vi "Init_Calculation.vi"(8 "Tester Parameter":dbl[](array[numeric]), 9 "DDM Parameter":dbl[](array[numeric])) -> (2 "Data":dbl[](array[numeric]))   [LabVIEW 2017]
panel:
  out "voltage":dbl
  out "current":dbl
  out "power":dbl
  out "Ambient pressure":dbl
  out "Ambient temperature":dbl
  out "Ambient humidity":dbl
  out "pressure":dbl
  out "power":dbl
  out "speed":dbl
  out "power":dbl
  out "current":dbl
  out "voltage":dbl
  out "delta_v":dbl
  out "ddm real power":dbl
  out "DDM_Pressure corrected":dbl
  # "Suction Power at Rated Power [AW]"
  # "Measured Volumetric Flow Rate (Q)"
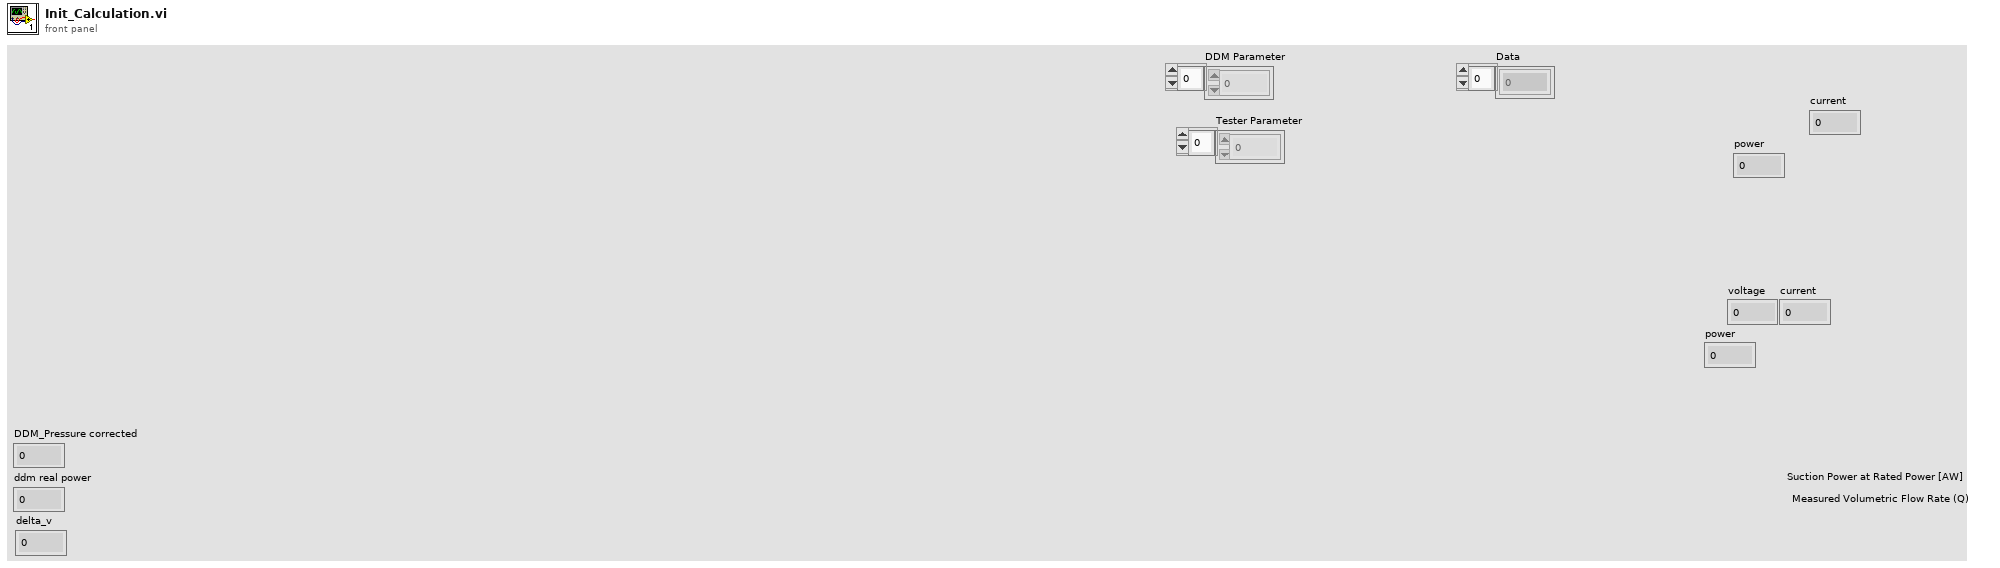
[diagram p1: front panel]
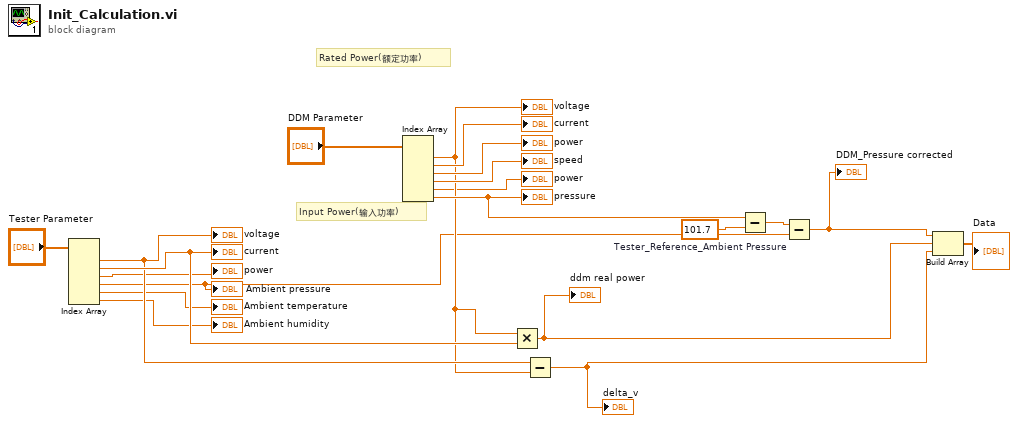
[diagram p0: block diagram]
diagram:
  w20 = 101.7  # Tester_Reference_Ambient Pressure
  # "Input Power(输入功率)"
  # "Rated Power(额定功率)"
  n1 = Index Array(array="Tester Parameter") -> (element #1=w11:dbl, element #2=w12:dbl, element #3=→"power":dbl, element #4=w9:dbl, element #5=→"Ambient temperature":dbl, element #6=→"Ambient humidity":dbl)  [unwired: 6 in]
  "voltage" <- w11
  "current" <- w12
  "Ambient pressure" <- w9
  n2 = Index Array(array="DDM Parameter") -> (element #1=w10:dbl, element #2=→"current":dbl, element #3=→"power":dbl, element #4=→"speed":dbl, element #5=→"power":dbl, element #6=w13:dbl)  [unwired: 6 in]
  "voltage" <- w10
  "pressure" <- w13
  n3 = Multiply(x=w10, y=w12) -> (x*y=w3:dbl)
  "ddm real power" <- w3
  n4 = Subtract(x=w11, y=w10) -> (x-y=w2:dbl)
  "delta_v" <- w2
  n5 = Subtract(x=w13, y=w20) -> (x-y=w19:dbl)
  n6 = Subtract(x=w19, y=w9) -> (x-y=w4:dbl)
  "DDM_Pressure corrected" <- w4
  n7 = Build Array(w4, w3, w2) -> (→"Data":dbl[])
